vi "Initial Picture.vi"(6 "error in (no error)":errorcluster, 8 "Pass":i32, 9 "fail":i32, 10 "中心位置":T1={"Cent X"=273.0, "Cent Y"=255.0, "Big1 R"=250.0, "Small1 R"=170.0, "Big2 R"=150.0, "Small2 R"=70.0, "Start_OutSide"=5.0, "Start_InSide"=9.0} {"Start_InSide" min=0.1 max=180.0; "Start_OutSide" min=0.1 max=180.0}, 11 "Image In":T2(plugin-control)) -> (0 "pass":string, 1 "fail":string, 3 "Image Out":T2(plugin-control), 4 "error out":errorcluster)   [LabVIEW 2017]
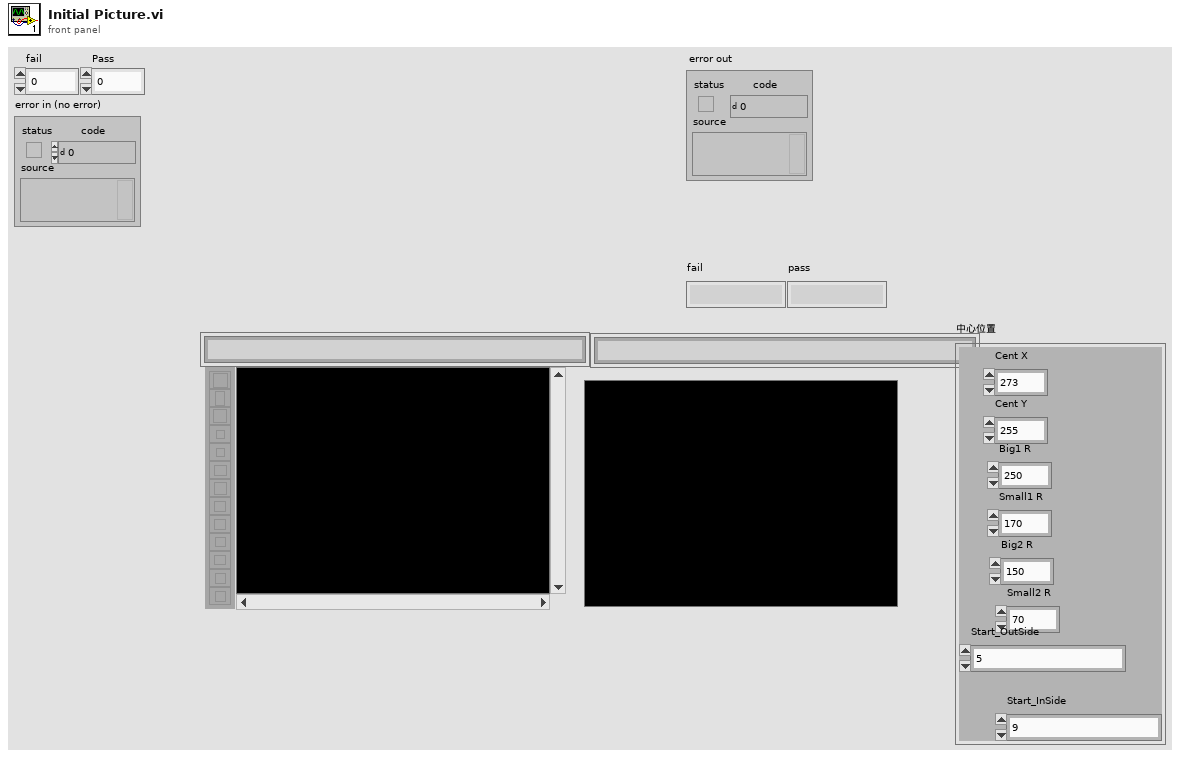
[diagram p1: front panel]
types:
  T1 = cluster{"Cent X":dbl, "Cent Y":dbl, "Big1 R":dbl, "Small1 R":dbl, "Big2 R":dbl, "Small2 R":dbl, "Start_OutSide":dbl, "Start_InSide":dbl}
  T2 = typedef "IMAQ Image.ctl" = refnum<image>
  T3 = cluster{"Left":i32, "Top":i32, "Right":i32, "Bottom":i32}
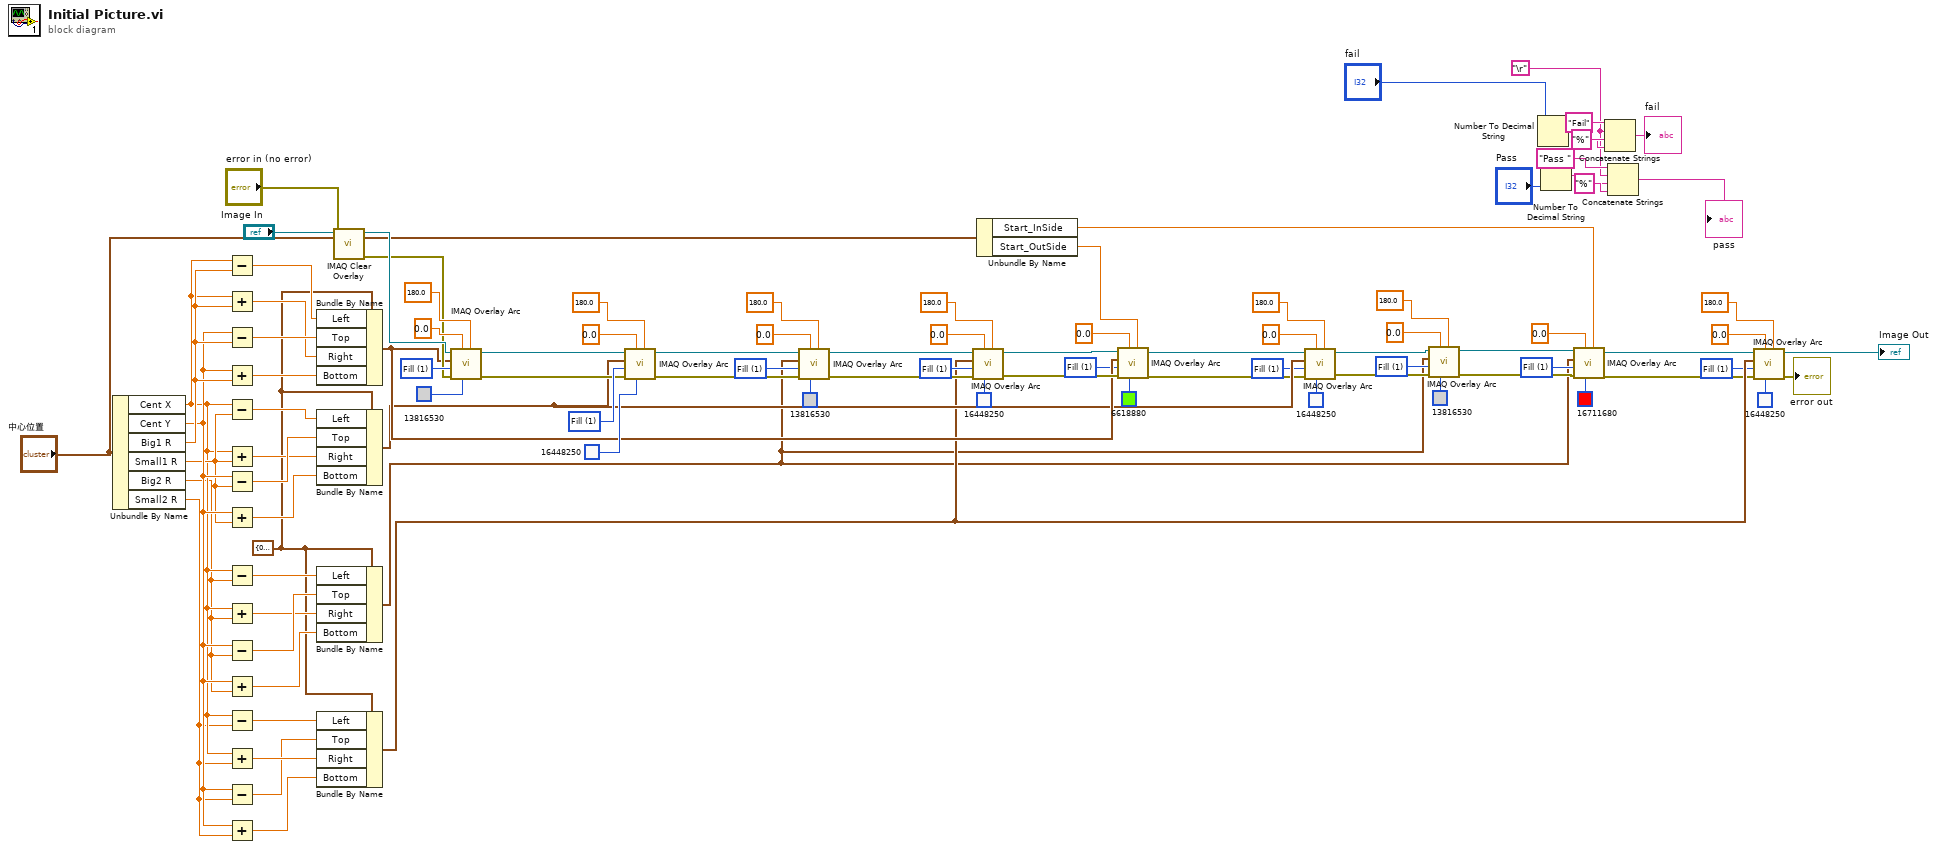
[diagram p0: block diagram]
diagram:
  w5 = "\r"
  w24 = u32 1 items=["Frame", "Fill"] ("Drawing Mode (Frame)")
  w31 = u32 1 items=["Frame", "Fill"] ("Drawing Mode (Frame)")
  w27 = u32 1 items=["Frame", "Fill"] ("Drawing Mode (Frame)")
  w38 = u32 1 items=["Frame", "Fill"] ("Drawing Mode (Frame)")
  w42 = u32 1 items=["Frame", "Fill"] ("Drawing Mode (Frame)")
  w69 = u32 1 items=["Frame", "Fill"] ("Drawing Mode (Frame)")
  w75 = u32 1 items=["Frame", "Fill"] ("Drawing Mode (Frame)")
  w51 = T3 {"Left"=0, "Top"=0, "Right"=0, "Bottom"=0} ("Bounding Rectangle")
  w92 = u32 1 items=["Frame", "Fill"] ("Drawing Mode (Frame)")
  w95 = u32 1 items=["Frame", "Fill"] ("Drawing Mode (Frame)")
  n1 = Unbundle By Name("中心位置") -> ("Cent X"=w54:dbl, "Cent Y"=w56:dbl, "Big1 R"=w77:dbl, "Small1 R"=w55:dbl, "Big2 R"=w53:dbl, "Small2 R"=w52:dbl)
  n2 = Subtract(x=w54, y=w77) -> (x-y=w85:dbl)
  n3 = Add(x=w54, y=w77) -> (x+y=w83:dbl)
  n4 = Subtract(x=w56, y=w77) -> (x-y=w84:dbl)
  n5 = Add(x=w56, y=w77) -> (x+y=w82:dbl)
  n6 = Subtract(x=w54, y=w55) -> (x-y=w81:dbl)
  n7 = Add(x=w54, y=w55) -> (x+y=w79:dbl)
  n8 = Subtract(x=w56, y=w55) -> (x-y=w80:dbl)
  n9 = Add(x=w56, y=w55) -> (x+y=w78:dbl)
  n10 = Subtract(x=w54, y=w53) -> (x-y=w64:dbl)
  n11 = Add(x=w54, y=w53) -> (x+y=w62:dbl)
  n12 = Subtract(x=w56, y=w53) -> (x-y=w63:dbl)
  n13 = Add(x=w56, y=w53) -> (x+y=w61:dbl)
  n14 = Subtract(x=w54, y=w52) -> (x-y=w57:dbl)
  n15 = Add(x=w54, y=w52) -> (x+y=w59:dbl)
  n16 = Subtract(x=w56, y=w52) -> (x-y=w58:dbl)
  n17 = Add(x=w56, y=w52) -> (x+y=w60:dbl)
  n18 = Bundle By Name(cluster=w51, "Left"=w85, "Top"=w84, "Right"=w83, "Bottom"=w82) -> (w46:T3)
  n19 = Bundle By Name(cluster=w51, "Left"=w81, "Top"=w80, "Right"=w79, "Bottom"=w78) -> (w45:T3)
  n20 = Bundle By Name(cluster=w51, "Left"=w64, "Top"=w63, "Right"=w62, "Bottom"=w61) -> (w17:T3)
  n21 = Bundle By Name(cluster=w51, "Left"=w57, "Top"=w58, "Right"=w59, "Bottom"=w60) -> (w44:T3)
  n22 = call "IMAQ Clear Overlay"("error in (no error)"="error in (no error)", "Image"="Image In") -> ("error out"=w50:errorcluster, "Image Out"=w86:T2)  [unwired: 8 in]
  n23 = call "IMAQ Overlay Arc"("End Angle (degrees)"=180.0, "Color"=u32 13816530, "Start Angle (degrees)"=0.0, "error in (no error)"=w50, "Drawing Mode (Frame)"=w95, "Bounding Rectangle"=w46, "Image"=w86) -> ("error out"=w88:errorcluster, "Image Out"=w89:T2)  [unwired: 3 in]
  n24 = call "IMAQ Overlay Arc"("End Angle (degrees)"=180.0, "Color"=u32 16448250, "Start Angle (degrees)"=0.0, "error in (no error)"=w88, "Drawing Mode (Frame)"=w92, "Bounding Rectangle"=w45, "Image"=w89) -> ("error out"=w65:errorcluster, "Image Out"=w72:T2)  [unwired: 3 in]
  n25 = call "IMAQ Overlay Arc"("End Angle (degrees)"=180.0, "Color"=u32 13816530, "Start Angle (degrees)"=0.0, "error in (no error)"=w65, "Drawing Mode (Frame)"=w75, "Bounding Rectangle"=w17, "Image"=w72) -> ("error out"=w66:errorcluster, "Image Out"=w67:T2)  [unwired: 3 in]
  n26 = call "IMAQ Overlay Arc"("End Angle (degrees)"=180.0, "Color"=u32 16448250, "Start Angle (degrees)"=0.0, "error in (no error)"=w66, "Drawing Mode (Frame)"=w69, "Bounding Rectangle"=w44, "Image"=w67) -> ("error out"=w48:errorcluster, "Image Out"=w49:T2)  [unwired: 3 in]
  n27 = Unbundle By Name("中心位置") -> ("Start_InSide"=w15:dbl, "Start_OutSide"=w16:dbl)
  n28 = call "IMAQ Overlay Arc"("End Angle (degrees)"=w16, "Color"=u32 6618880, "Start Angle (degrees)"=0.0, "error in (no error)"=w48, "Drawing Mode (Frame)"=w42, "Bounding Rectangle"=w46, "Image"=w49) -> ("error out"=w35:errorcluster, "Image Out"=w36:T2)  [unwired: 3 in]
  n29 = call "IMAQ Overlay Arc"("End Angle (degrees)"=180.0, "Color"=u32 16448250, "Start Angle (degrees)"=0.0, "error in (no error)"=w35, "Drawing Mode (Frame)"=w38, "Bounding Rectangle"=w45, "Image"=w36) -> ("error out"=w20:errorcluster, "Image Out"=w21:T2)  [unwired: 3 in]
  n30 = call "IMAQ Overlay Arc"("End Angle (degrees)"=180.0, "Color"=u32 13816530, "Start Angle (degrees)"=0.0, "error in (no error)"=w20, "Drawing Mode (Frame)"=w24, "Bounding Rectangle"=w17, "Image"=w21) -> ("error out"=w19:errorcluster, "Image Out"=w18:T2)  [unwired: 3 in]
  n31 = Number To Decimal String(number="fail") -> (decimal integer string=w14:string)  [unwired: 1 in]
  n32 = Number To Decimal String(number="Pass") -> (decimal integer string=w11:string)  [unwired: 1 in]
  n33 = call "IMAQ Overlay Arc"("End Angle (degrees)"=w15, "Color"=u32 16711680, "Start Angle (degrees)"=0.0, "error in (no error)"=w19, "Drawing Mode (Frame)"=w27, "Bounding Rectangle"=w17, "Image"=w18) -> ("error out"=w34:errorcluster, "Image Out"=w33:T2)  [unwired: 3 in]
  n34 = Concatenate Strings("Fail" ("字符串"), w5, w14, "%" ("字符串")) -> (→"fail":string)
  n35 = Concatenate Strings("Pass " ("字符串"), w5, w11, "%" ("字符串")) -> (→"pass":string)
  n36 = call "IMAQ Overlay Arc"("End Angle (degrees)"=180.0, "Color"=u32 16448250, "Start Angle (degrees)"=0.0, "error in (no error)"=w34, "Drawing Mode (Frame)"=w31, "Bounding Rectangle"=w44, "Image"=w33) -> ("error out"=→"error out":errorcluster, "Image Out"=→"Image Out":T2)  [unwired: 3 in]
